vi "Check.vi"(8 "error in (no error)":errorcluster, 11 "FPT_SParam_Switching in":refnum<class "FPT_SParam_Switching.lvclass">) -> (0 "error out":errorcluster, 3 "FPT_SParam_Switching out":refnum<class "FPT_SParam_Switching.lvclass">)   [LabVIEW 2023, in "FPT_SParam_Switching.lvclass"]
uses:
  FPT_SParam_Switching.lvclass
  FPT_SParam_Switching.lvclass/FPT_SParam_Switching.ctl
  <vilib>/niSPML/S-parameters/S-Parameters.lvlib
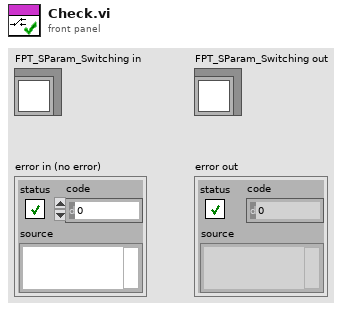
[diagram p1: front panel]
types:
  T1 = typedef "niSwitch Path Capability.ctl" = i32
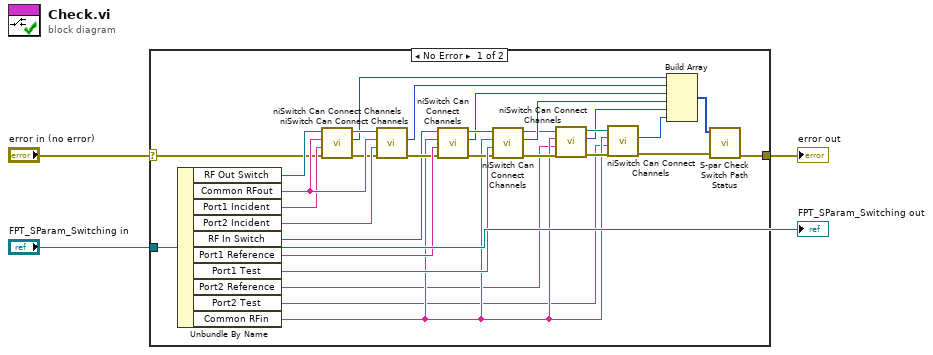
[diagram p0: block diagram]
diagram:
  n1 = case shown="No Error" "error in (no error)" {
    selector: "error in (no error)" -> [w27 w34]
    tunnel: "FPT_SParam_Switching in" -> [w26 _]
    tunnel: [w7 w34] -> w3
    frame No Error {
      n2 = Unbundle By Name(w26) -> ("RF Out Switch"=w28:refnum<k15>, "Common RFout"=w33:string, "Port1 Incident"=w32:string, "Port2 Incident"=w31:string, "RF In Switch"=w15:refnum<k15>, "Port1 Reference"=w30:string, "Port1 Test"=w29:string, "Port2 Reference"=w5:string, "Port2 Test"=w4:string, "Common RFin"=w6:string)
      n3 = call <instrlib>:"niSwitch Can Connect Channels.vi"("error in (no error)"=w27, "channel 2"=w32, "channel 1"=w33, "instrument handle"=w28) -> ("error out"=w25:errorcluster, "path capability"=w20:T1, "instrument handle out"=w24:refnum<k15>)  [unwired: 5 in]
      n4 = call <instrlib>:"niSwitch Can Connect Channels.vi"("error in (no error)"=w25, "channel 2"=w31, "channel 1"=w33, "instrument handle"=w24) -> ("error out"=w23:errorcluster, "path capability"=w19:T1)  [unwired: 5 in, 1 out]
      n5 = call <instrlib>:"niSwitch Can Connect Channels.vi"("error in (no error)"=w23, "channel 2"=w30, "channel 1"=w6, "instrument handle"=w15) -> ("error out"=w22:errorcluster, "path capability"=w18:T1, "instrument handle out"=w21:refnum<k15>)  [unwired: 5 in]
      n6 = call <instrlib>:"niSwitch Can Connect Channels.vi"("error in (no error)"=w22, "channel 2"=w29, "channel 1"=w6, "instrument handle"=w21) -> ("error out"=w14:errorcluster, "path capability"=w17:T1, "instrument handle out"=w13:refnum<k15>)  [unwired: 5 in]
      n7 = call <instrlib>:"niSwitch Can Connect Channels.vi"("error in (no error)"=w14, "channel 2"=w5, "channel 1"=w6, "instrument handle"=w13) -> ("error out"=w12:errorcluster, "path capability"=w9:T1, "instrument handle out"=w11:refnum<k15>)  [unwired: 5 in]
      n8 = call <instrlib>:"niSwitch Can Connect Channels.vi"("error in (no error)"=w12, "channel 2"=w4, "channel 1"=w6, "instrument handle"=w11) -> ("error out"=w10:errorcluster, "path capability"=w8:T1)  [unwired: 5 in, 1 out]
      n9 = Build Array(w20, w19, w18, w17, w9, w8) -> (w16:T1[])
      n10 = call <vilib>:"S-par Check Switch Path Status.vi"("error in (no error)"=w10, "Path status"=w16) -> ("error out"=w7:errorcluster)  [unwired: 9 in]
    }
    frame Error {
    }
  }
  "error out" <- w3
  "FPT_SParam_Switching out" <- "FPT_SParam_Switching in"
